vi "Update Observers.vi"(8 "error in":errorcluster, 11 "GUI Facade in":refnum<class "GUI Facade.lvclass">) -> (0 "error out":errorcluster, 3 "GUI Facade out":refnum<class "GUI Facade.lvclass">)   [LabVIEW 2018, in "GUI Facade.lvclass"]
uses:
  GUI Facade.lvclass
  Observer/Data Subject.lvclass
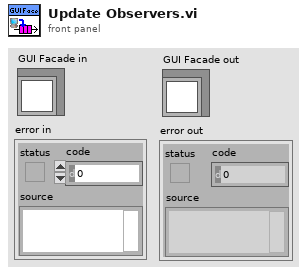
[diagram p1: front panel]
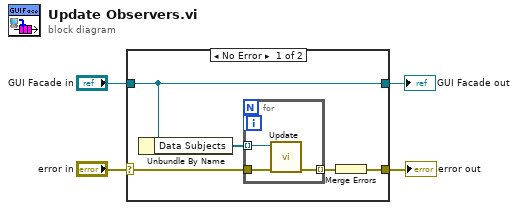
[diagram p0: block diagram]
diagram:
  n1 = case shown="No Error" "error in" {
    selector: "error in" -> [w7 w14]
    tunnel: [w5 w14] -> w3
    tunnel: [w9 w13] -> w1
    tunnel: "GUI Facade in" -> [w9 w13]
    frame No Error {
      n2 = Unbundle By Name(w9) -> ("Data Subjects"=w8:refnum<class "Data Subject.lvclass">[])
      n3 = for {
        workers-P: _ -> [_]
        tunnel: w8 -> [w12] mode=indexing
        tunnel: w7 -> [w11]
        tunnel: [w10] -> w6 mode=indexing
        n4 = call-dynamic "Update.vi"("error in"=w11, "Data Subject in"=w12) -> ("error out"=w10:errorcluster)  [unwired: 7 in, 2 out]
      }
      n5 = Merge Errors(w6) -> (w5:errorcluster)
    }
    frame Error {
    }
  }
  "error out" <- w3
  "GUI Facade out" <- w1
